vi "Set Minimum Log Level.vi"(8 "error in (no error)":errorcluster, 10 "log level (Info)":T1=enum."Info", 11 "name (\"Default\")":string="Default") -> (0 "error out":errorcluster)   [LabVIEW 2018, in "GLog.lvlib"]
doc: "Set the minimum log level of a specific logger in the Registry by name.\n\nIf the name provided does not match any currently registered loggers, this VI will return an error."
uses:
  GLog.lvlib
  Log Levels.ctl
  registry/Registry.lvlib
panel:
  # "Connector Pane"
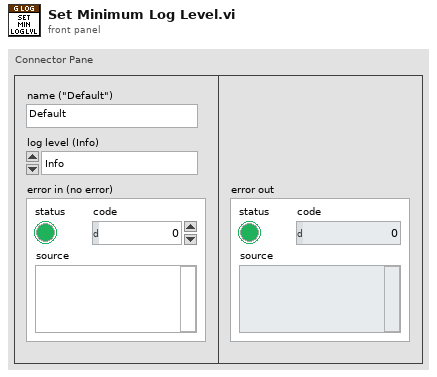
[diagram p1: front panel]
types:
  T1 = typedef "GLog.lvlib/Log Levels.ctl" = enum16{"Trace", "Debug", "Info", "Warning", "Error", "Critical"}
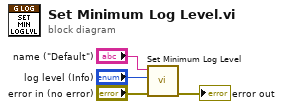
[diagram p0: block diagram]
diagram:
  n1 = call "Set Minimum Log Level.vi"("error in (no error)"="error in (no error)", "log level"="log level (Info)", "logger name"="name (\"Default\")") -> ("error out"=→"error out":errorcluster)  [unwired: 8 in]
